vi "Vector_add.vi"(11 "vectors":T1[](array[typedef])=[{"vector"={"length"=30.0, "angle"=45.0, "sense"=FALSE}, "color"=0, "offset"={"X origin"=0, "Y origin"=0}}, {"vector"={"length"=70.0, "angle"=10.0, "sense"=FALSE}, "color"=16722176, "offset"={"X origin"=36, "Y origin"=60}}, {"vector"={"length"=30.0, "angle"=-15.0, "sense"=FALSE}, "color"=46165, "offset"={"X origin"=58, "Y origin"=18}}] {"offset"."Y origin" scale=0.0..100.0; "offset"."X origin" scale=0.0..100.0; "vector"."length" format="%.1f"; "vector"."angle" format="%.1f"}) -> (3 "vectors":T1[](array[typedef])=[{"vector"={"length"=30.0, "angle"=45.0, "sense"=FALSE}, "color"=0, "offset"={"X origin"=0, "Y origin"=0}}, {"vector"={"length"=70.0, "angle"=10.0, "sense"=FALSE}, "color"=16722176, "offset"={"X origin"=36, "Y origin"=60}}, {"vector"={"length"=30.0, "angle"=-15.0, "sense"=FALSE}, "color"=46165, "offset"={"X origin"=58, "Y origin"=18}}] {"offset"."Y origin" scale=0.0..100.0; "offset"."X origin" scale=0.0..100.0; "vector"."length" format="%.1f"; "vector"."angle" format="%.1f"})   [LabVIEW 2024]
uses:
  Vector_typedef.ctl
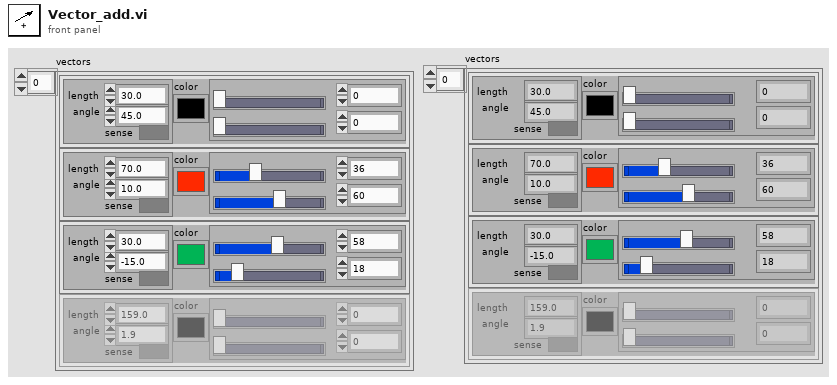
[diagram p1: front panel]
types:
  T1 = typedef "Vector_typedef.ctl" = cluster{"vector":cluster{"length":dbl, "angle":dbl, "sense":bool}, "color":u32, "offset":cluster{"X origin":i16, "Y origin":i16}}
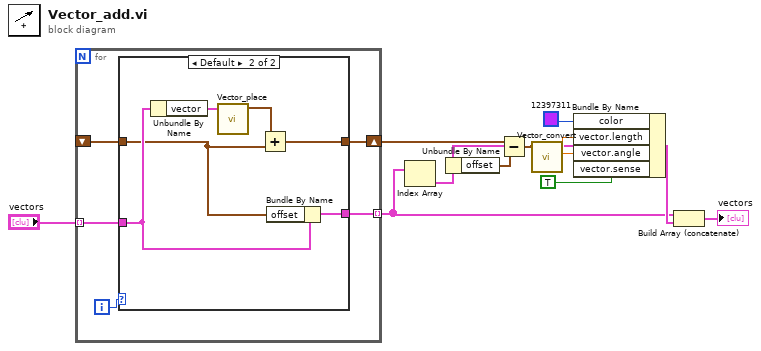
[diagram p0: block diagram]
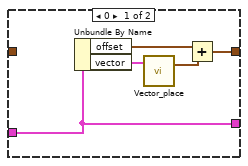
[diagram p2: hidden frame]
diagram:
  n1 = for {
    tunnel: "vectors" -> [w17] mode=indexing
    tunnel: [w16] -> w4 mode=indexing
    shift-right: [w15] -> w11
    shift-left: _ -> [w14]
    i -> [w13]
    n2 = case shown="Default" w13 {
      tunnel: w17 -> [w21 w25]
      tunnel: [w21 w24] -> w16
      tunnel: [w18 w27] -> w15
      tunnel: w14 -> [_ w23]
      frame 0 {
        n3 = Unbundle By Name(w21) -> ("offset"=w20:cluster{"X origin":i16, "Y origin":i16}, "vector"=w22:cluster{"length":dbl, "angle":dbl, "sense":bool})
        n4 = call "Vector_place.vi"("vector"=w22) -> ("x,y"=w19:cluster{dbl, dbl})  [unwired: 10 in]
        n5 = Add(x=w20, y=w19) -> (x+y=w18:cluster{dbl, dbl})
      }
      frame Default {
        n6 = Unbundle By Name(w25) -> ("vector"=w28:cluster{"length":dbl, "angle":dbl, "sense":bool})
        n7 = call "Vector_place.vi"("vector"=w28) -> ("x,y"=w26:cluster{dbl, dbl})  [unwired: 10 in]
        n8 = Add(x=w26, y=w23) -> (x+y=w27:cluster{dbl, dbl})
        n9 = Bundle By Name(cluster=w25, "offset"=w23) -> (w24:T1)
      }
    }
  }
  n10 = Index Array(array=w4) -> (element=w3:T1)  [unwired: 1 in]
  n11 = Unbundle By Name(w3) -> ("offset"=w2:cluster{"X origin":i16, "Y origin":i16})
  n12 = Subtract(x=w11, y=w2) -> (x-y=w10:cluster{dbl, dbl})
  n13 = call "Vector_convert.vi"("x,y"=w10) -> ("angle"=w9:dbl, "mag"=w8:dbl)  [unwired: 9 in]
  n14 = Bundle By Name(cluster=w3, "color"=u32 12397311, "vector.length"=w8, "vector.angle"=w9, "vector.sense"=TRUE) -> (w6:T1)
  n15 = Build Array (concatenate)(w4, w6) -> (→"vectors":T1[])
